vi "Local Json Pretty Formatter.vi"(8 "error in":errorcluster, 10 "data name in":string, 11 "json in":string) -> (0 "error out":errorcluster, 3 "json out":string)   [LabVIEW 2022 SP3]
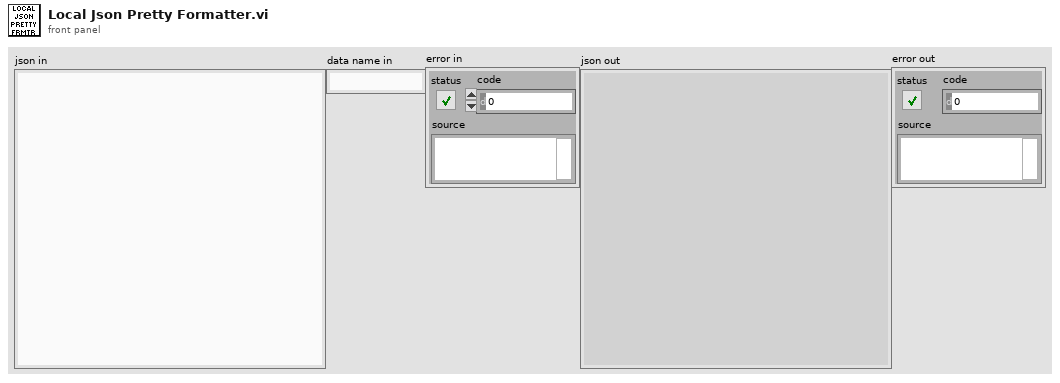
[diagram p1: front panel]
types:
  T1 = typedef "ATS Framework Fields.ctl" = cluster{"data name":string, "tools path":string, "scripts path":string}
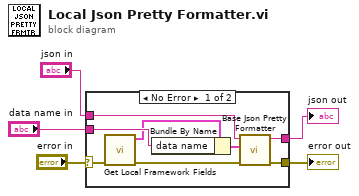
[diagram p0: block diagram]
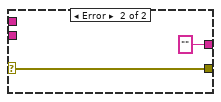
[diagram p2: hidden frame]
diagram:
  n1 = case shown="No Error" "error in" {
    selector: "error in" -> [w10 w15]
    tunnel: [w13 w15] -> w5
    tunnel: [w12 "" ("json out")] -> w4
    tunnel: "data name in" -> [w9 _]
    tunnel: "json in" -> [w6 _]
    frame No Error {
      n2 = call "Get Local Framework Fields.vi"("error in"=w10) -> ("error out"=w11:errorcluster, "ATS Framework Fields out"=w8:T1)  [unwired: 9 in]
      n3 = Bundle By Name(cluster=w8, "data name"=w9) -> (w7:T1)
      n4 = call "Base Json Pretty Formatter.vi"("error in"=w11, "ATS Framework Fields in"=w7, "json in"=w6) -> ("error out"=w13:errorcluster, "json out"=w12:string)  [unwired: 7 in]
    }
    frame Error {
    }
  }
  "error out" <- w5
  "json out" <- w4
